vi "analogReadCustom.vi"() -> ()   [LabVIEW 2013]
doc: "This example demonstrates how to read N channels of analog input from a LINX device."
uses:
  <vilib>/MakerHub/LINX/Private/Type Defs/User Platform.ctl
  <vilib>/MakerHub/LINX/Private/Type Defs/Interface.ctl
  <vilib>/MakerHub/LINX/Public/Peripherals/Analog/Analog Read N Chans.vi
  <vilib>/MakerHub/LINX/Private/Local IO/LinxAnalogRead.vi
  <vilib>/MakerHub/LINX/Public/Utilities/Check Channel.vi
  <vilib>/MakerHub/LINX/Private/Utilties/Generate Error.vi
  <vilib>/MakerHub/LINX/LMH-LINX.lvlib
panel:
  out "Displacement":u32(slide) scale=0.0..100.0
  out "Load Cell Force":dbl(knob) scale=0.0..10.0
  out "Output  RPM":dbl(knob) scale=0.0..10.0
  out "Input RPM":dbl(knob) scale=0.0..10.0
  in  "Serial Port":refnum<visa-resource-name>="N/A"
  in  "Baud Rate Override":u32=115200
  in  "Stop Button":bool
  out "Loop Rate (Hz)":u32
  # "Instructions:\n1) Select COM Port\n3) Click the run arrow (top left)\n4) Press the stop button when finished"
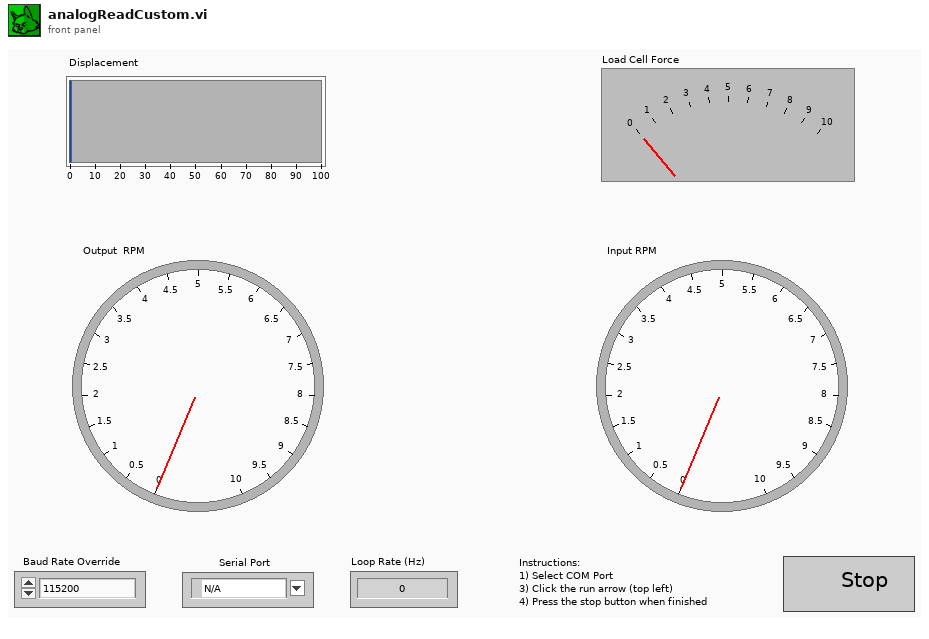
[diagram p1: front panel]
types:
  T1 = typedef "LMH-LINX.lvlib/Interface.ctl" = enum16{"Serial", "TCP"}
  T2 = typedef "LMH-LINX.lvlib/User Platform.ctl" = enum16{"Default", "Remote", "Local"}
  T3 = typedef "LMH-LINX.lvlib/LINX Ref.ctl" = cluster{"IO":T4, "Interface":T1, "LINX Device Config":T5}
  T4 = typedef "LMH-LINX.lvlib/Platform.ctl" = enum16{"Remote", "Local"}
  T5 = typedef "LMH-LINX.lvlib/Device.lvlib/LINX Device Config.ctl" = cluster{"Interface":T1, "COM Port":refnum<visa-resource-name>, "TCP Configuration":T6, "Device Family":u8, "Device ID":u8, "Device Name":string, "TCP Ref":refnum<k5>, "Channels":T7}
  T6 = typedef "LMH-LINX.lvlib/Device.lvlib/TCP Config.ctl" = cluster{"IP Address":string, "Port":u16}
  T7 = typedef "LMH-LINX.lvlib/Channels.ctl" = cluster{"DI":u8[], "DO":u8[], "AI":u8[], "AO":u8[], "PWM":u8[], "QE":u8[], "UART":u8[], "I2C 2":u8[], "SPI":u8[], "CAN":u8[], "Servo":u8[], "AI Ref (V)":dbl, "AI Resolution (Bits)":u8, "AO Ref (V)":dbl, "AO Resolution (Bits)":u8}
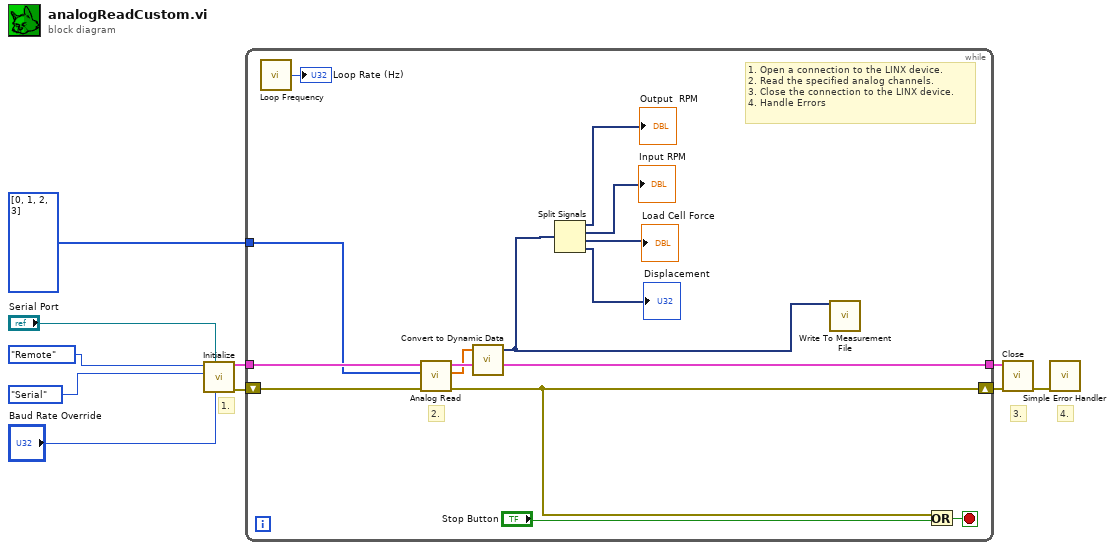
[diagram p0: block diagram]
diagram:
  # "4."
  # "3."
  # "1."
  n1 = call <vilib>:"Initialize.vi"("Baud Rate Override"="Baud Rate Override", "Serial Port"="Serial Port", "Interface"=Interface."Serial", "IO"=User_Platform."Remote" ("Platform")) -> ("Error Out"=w2:errorcluster, "LINX Resource"=w3:T3)  [unwired: 5 in, 1 out]
  n2 = while {
    tunnel: w3 -> [w19]
    tunnel: [w24] -> w10
    shift-right: [w21] -> w9
    shift-left: w2 -> [w18]
    tunnel: u8[] [0, 1, 2, 3] ("AI Channel(s)") -> [w13]
    stop <- w23 stop-if-true
    # "1. Open a connection to the LINX device.\n2. Read the specified analog channels.\n3. Close the connection to the LINX device.\n4. Handle Errors"
    # "2."
    n3 = call <vilib>:"Loop Frequency.vi"() -> ("Loop Rate (Hz)"=→"Loop Rate (Hz)":u32)
    n4 = call-poly <vilib>:"Analog Read.vi"("Error In"=w18, "AI Channel(s)"=w13, "LINX Resource"=w19) -> ("Error Out"=w21:errorcluster, "Voltages"=w12:dbl[], "LINX Resource"=w24:T3)  [unwired: 5 in, 1 out]
    n5 = call "Convert to Dynamic Data"("Array"=w12) -> ("Dynamic Data Type"=w11:dynamicdata)  [unwired: 3 in]
    n6 = Split Signals(w11) -> (→"Output  RPM":dynamicdata, →"Input RPM":dynamicdata, →"Load Cell Force":dynamicdata, →"Displacement":dynamicdata)  [unwired: 4 in]
    n7 = call "Write To Measurement File"("Signals"=w11) -> ()  [unwired: 16 in, 3 out]
    n8 = Or(x=w21, y="Stop Button") -> (x .or. y?=w23:bool)
  }
  n9 = call <vilib>:"Close.vi"("Error In"=w9, "LINX Resource"=w10) -> ("Error Out"=w8:errorcluster)  [unwired: 9 in]
  n10 = call <vilib>:"Simple Error Handler.vi"("error in (no error)"=w8) -> ()  [unwired: 4 in, 5 out]
